vi "Compiled Help Menu Wizard.vi"   [LabVIEW 2015]
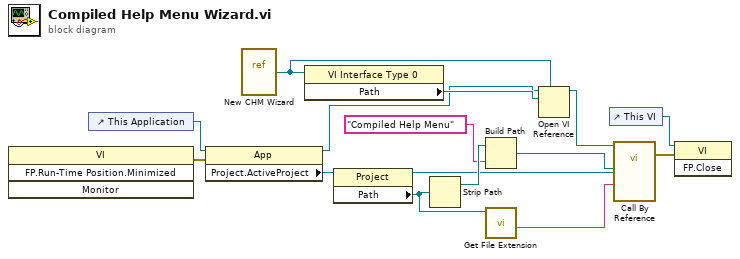
[diagram p0: block diagram]
diagram:
  n1 = invoke class="VI" method="FP.Run-Time Position.Minimized"() -> (error out=w8:errorcluster)  [unwired: 4 in, 3 out]
  n2 = control-ref of="This Application"() -> (w15:refnum<vi>)
  n3 = property class="App"(reference=w15, error in=w8) -> (reference out=w3:refnum<vi>, "Project.ActiveProject"=w14:refnum<vi>)  [unwired: 1 out]
  n4 = vi-ref "New CHM Wizard.vi"() -> (w1:refnum<vi>)
  n5 = property class="VI Interface Type 0"(reference=w1) -> ("Path"=w4:path)  [unwired: 1 in, 2 out]
  n6 = property class="Project"(reference=w14) -> (reference out=w5:refnum<vi>, "Path"=w7:path)  [unwired: 1 in, 1 out]
  n7 = Strip Path(path=w7) -> (stripped path=w13:path)  [unwired: 1 out]
  n8 = Build Path(base path=w13, name or relative path="Compiled Help Menu") -> (appended path=w11:path)
  n9 = call <vilib>:"Get File Extension.vi"("file"=w7) -> ("filename without extension"=w6:string)  [unwired: 6 in, 4 out]
  n10 = Open VI Reference(type specifier VI Refnum (for type only)=w1, application reference (local)=w3, vi path=w4) -> (vi reference=w2:refnum<vi>)  [unwired: 3 in, 1 out]
  n11 = control-ref of="This VI"() -> (w10:refnum<vi>)
  n12 = call-by-ref "?"(reference=w2, "Project:Active Project"=w5, "Title"=w6, "Base CHM Directory"=w11) -> (error out=w9:errorcluster)  [unwired: 10 in, 1 out]
  n13 = invoke class="VI" method="FP.Close"(reference=w10, error in=w9) -> ()  [unwired: 1 in, 3 out]
